vi "Create from SQL Values.vi"(8 "error in (no error)":errorcluster, 11 "recordset data":variant[](array[variant])) -> (0 "error out":errorcluster, 3 "Expense Summary out":refnum<class "Expense Summary.lvclass">)   [LabVIEW 2018, in "Expense Summary.lvclass"]
uses:
  Expense Summary.lvclass
  Expense Summary.lvclass/Expense Summary.ctl
  <vilib>/addons/database/NI_Database_API.lvlib
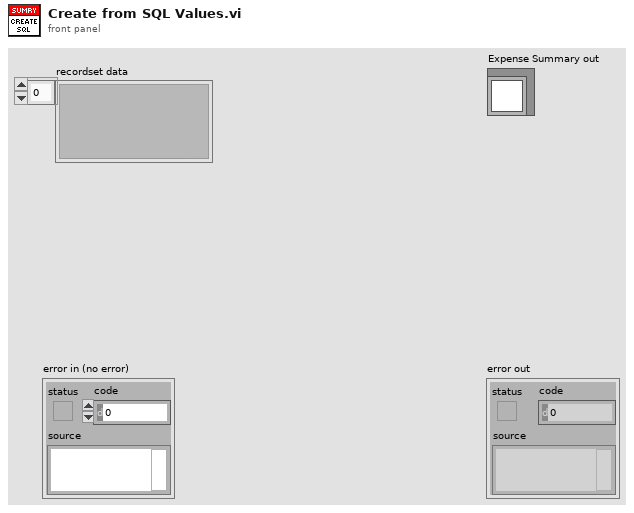
[diagram p1: front panel]
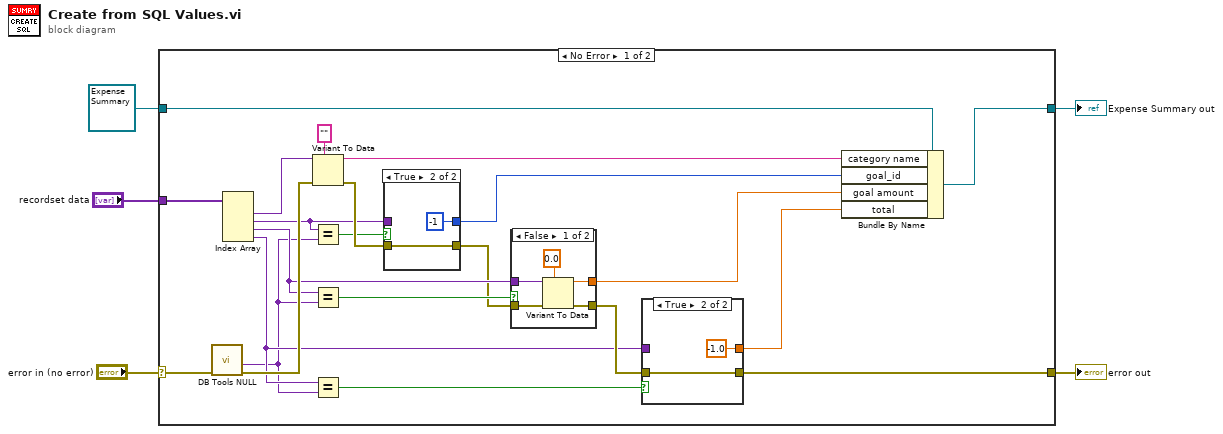
[diagram p0: block diagram]
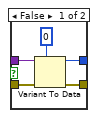
[diagram p2: hidden frame]
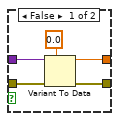
[diagram p3: hidden frame]
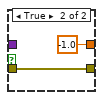
[diagram p4: hidden frame]
diagram:
  n1 = case shown="No Error" "error in (no error)" {
    selector: "error in (no error)" -> [w18 w50]
    tunnel: [w25 w50] -> w4
    tunnel: [w22 w49] -> w2
    tunnel: refnum<class "Expense Summary.lvclass"> refnum ("Expense Summary in") -> [w23 w49]
    tunnel: "recordset data" -> [w27 _]
    frame No Error {
      n2 = call <vilib>:"DB Tools NULL.vi"("error in (no error)"=w18) -> ("error out"=w17:errorcluster, "NULL"=w8:variant)  [unwired: 9 in]
      n3 = Index Array(array=w27) -> (element #1=w26:variant, element #2=w7:variant, element #3=w13:variant, element #4=w14:variant)  [unwired: 4 in]
      n4 = Variant To Data(error in=w17, type="", Variant=w26) -> (data=w20:string, error out=w11:errorcluster)
      n5 = Equal?(x=w7, y=w8) -> (x = y?=w6:bool)
      n6 = Equal?(x=w13, y=w8) -> (x = y?=w16:bool)
      n7 = Equal?(x=w14, y=w8) -> (x = y?=w15:bool)
      n8 = case shown="True" w6 {
        tunnel: w7 -> [w32 _]
        tunnel: w11 -> [w31 w34]
        tunnel: [w30 w34] -> w10
        tunnel: [w28 -1 ("goal_id")] -> w9
        frame False {
          n9 = Variant To Data(error in=w31, type=0 ("goal_id"), Variant=w32) -> (data=w28:i32, error out=w30:errorcluster)
        }
        frame True {
        }
      }
      n10 = case shown="False" w16 {
        tunnel: [w46 w47] -> w24
        tunnel: w10 -> [w45 w47]
        tunnel: [w43 -1.0] -> w12
        tunnel: w13 -> [w42 _]
        frame False {
          n11 = Variant To Data(error in=w45, type=0.0, Variant=w42) -> (data=w43:dbl, error out=w46:errorcluster)
        }
        frame True {
        }
      }
      n12 = case shown="True" w15 {
        tunnel: w14 -> [w39 _]
        tunnel: [w38 w41] -> w25
        tunnel: w24 -> [w37 w41]
        tunnel: [w36 -1.0] -> w19
        frame False {
          n13 = Variant To Data(error in=w37, type=0.0, Variant=w39) -> (data=w36:dbl, error out=w38:errorcluster)
        }
        frame True {
        }
      }
      n14 = Bundle By Name(cluster=w23, "category name"=w20, "goal_id"=w9, "goal amount"=w12, "total"=w19) -> (w22:refnum<class "Expense Summary.lvclass">)
    }
    frame Error {
    }
  }
  "error out" <- w4
  "Expense Summary out" <- w2
